vi "Publish Group.vi"(8 "error in (no error)":errorcluster, 10 "Group":refnum<class "Group.lvclass">, 11 "Module in":refnum<class "Module.lvclass">) -> (0 "error out":errorcluster, 3 "Module out":refnum<class "Module.lvclass">)   [LabVIEW 2020, in "Volatus.lvlib" / "Module.lvclass"]
uses:
  Module.lvclass
  lv-vecto/Vecto/Group/Group.lvclass
  Module.lvclass/Module.ctl
  VolatusAPI/VolatusAPI.lvclass/VolatusAPI.ctl
  lv-vecto/Vecto/Group/Group.lvclass/Group.ctl
  lv-vecto/Vecto/Group/Node.vi
  lv-vecto/Vecto/Group Config/Get Info.vi
  VolatusAPI/Publish to Local Subs.vi
  VolatusAPI/VolatusAPI.lvclass
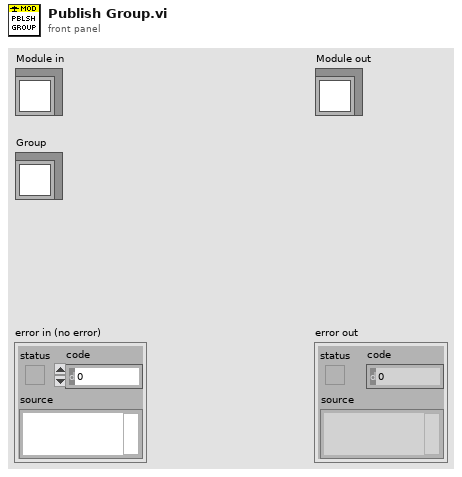
[diagram p1: front panel]
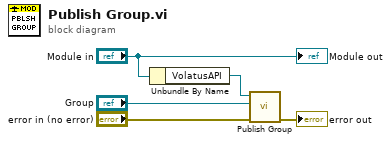
[diagram p0: block diagram]
diagram:
  n1 = Unbundle By Name("Module in") -> ("VolatusAPI"=w4:refnum<class "VolatusAPI.lvclass">)
  n2 = call "Publish Group.vi"("error in (no error)"="error in (no error)", "Group"="Group", "VolatusAPI in"=w4) -> ("error out"=→"error out":errorcluster)  [unwired: 7 in, 1 out]
  "Module out" <- "Module in"
